vi "high pass filter caller.vi"() -> ()   [LabVIEW 2014]
doc: "high pass filter caller BAE3\n\nDisplays a high pass filter as an Amplitude v. Time graph with a two-level signal [-1 or +1] controlled by a toggle switch.\n\nSubVi:\nITR HP BAE3\n\nBeverly Abadines\nPHY 350: E3"
panel:
  in  "corner period (steps)":dbl(slide)=100.00000000000004 scale=1.0..1000.0
  in  "Input Signal":bool
  in  "stop":bool
  out "Signal Monitor":cluster{dbl, dbl}(graph)={0.7537027844924145, 0.5116982465814583}
  # "High Pass Filter"
  # "Bever;y Abadines\nPHY 350\nE3"
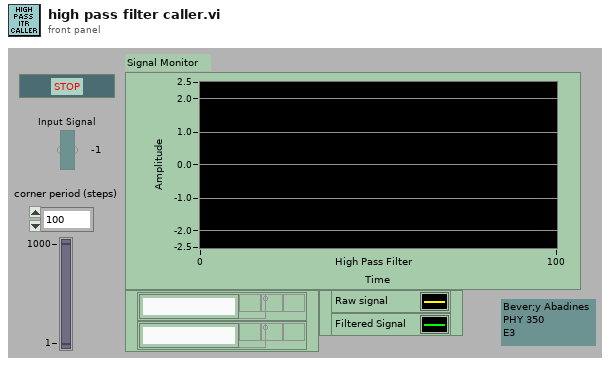
[diagram p1: front panel]
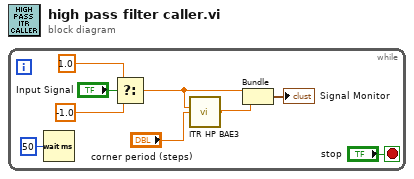
[diagram p0: block diagram]
diagram:
  n1 = while {
    stop <- "stop" stop-if-true
    n2 = Wait (ms)(milliseconds to wait=u32 50) -> ()  [unwired: 1 out]
    n3 = Select(t=1.0, s="Input Signal", f=-1.0) -> (s? t:f=w3:dbl)
    n4 = call "ITR HP BAE3.vi"("input"=w3, "T (corner period) [steps]"="corner period (steps)") -> ("output"=w5:dbl)  [unwired: 13 in]
    n5 = Bundle("f"=w3, "output"=w5) -> (→"Signal Monitor":cluster{"f":dbl, "output ":dbl})  [unwired: 1 in]
  }
